vi "读取SuperDog数据.vi"(8 "length":u32=128, 9 "offset":u32, 10 "fileid":u32=65524, 11 "feature_id":u32=1) -> (1 "buffer out(Hex)":string, 2 "license handle":u32)   [LabVIEW 2009]
uses:
  dog_windows_UCPBI.dll
panel:
  out "function return 2":i32
  out "out handle":u32
  in  "vendor_code":string="Ur6fPGYDEBkws3SZISCrIAjySjKgu+8CGpfZwvGywxzzFI7qfH5o4nn4T/VCSRk/BzHd89oLkO1FSQ6hEVYUq6gMbLM2C/cFM+If39OR5tb8bGFz9qR0CZDkjzzjmu7KkZUG/Iybd++jcPT1fCPTGl6yJQ63DfZrtajYZMbIcHXXH5GeLmq0E8DxHQfjk36CNBnpZp3ut4e1U62BwqZI8PukpzjI2GcYs99UUUsufQbOliL2dlPu5jsionzy4pNB7CtL1sNOSyL4lXeGzFITSf8f2PBTMx9pRbZVpRKcaSkgwkYIgZXZK4Mh7WJhSM9dVyuowWAwHAuS1RiQbUqLqNZTlQihipkbiFrvlvM/xVR66Srt2LVSqv6RGu0aWaNM+SeJAKQlu1FskQm2TRpYQAGcH9IYTi3NGin13cji+Dth8rVwEY04N9GmpGLG1KBZxXFIIYBy0O8uMggrvjMlMgu9vg/saWFb+shkOQnET6WxlanEW2MfoWqVm2hwmy6exQBR69dptwkQ5qXprYd3dqA3rTyUqz4W29XJ+nztSzZRMl1Jt8sxCVvSX0Lg7SiRSoedaijV3a2EegSPrw4xW5o7O+yQItLwaVks4udB3kVz+wOrOTrxlWOz3u5MHdUzWFHlrTQRDlt9xBAqO+PT5M85/8ZLpyxHHIIpvOqXtCxgrtKMy1SD3O6zMZutZlcCE6Gj9CK6vz9O5JlMBBA5bEYYZSUUACDo9z6fP/F0VUeEMhqr9wsmyQdBIlBGlYM0GsvXLcJNL74RPewQkgLEhWc4txMcn6l0ey6Ic+qXpypp1e5qgjwyVACyJgZphW3HVcmpmld71etpUP0WgIY7Uuso2ZTDXKwBoh4l7Q5ZiKurwwQ5USgmL+vGx1H60ANV7LAoiEM2/cAiuUL+fKvyTMrWDED5hSzclM+TYLwc2vTgNmcQwlUcbjKlJIQTYSpPLpAa7xsThJ34yY5WOoiQLQ=="
  out "function return":i32
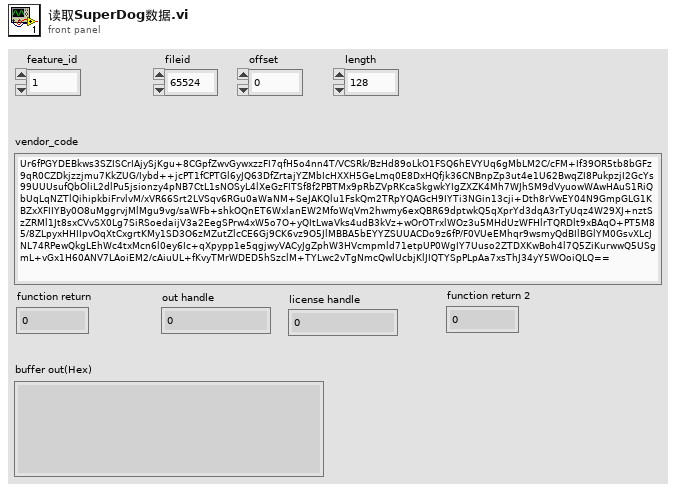
[diagram p1: front panel]
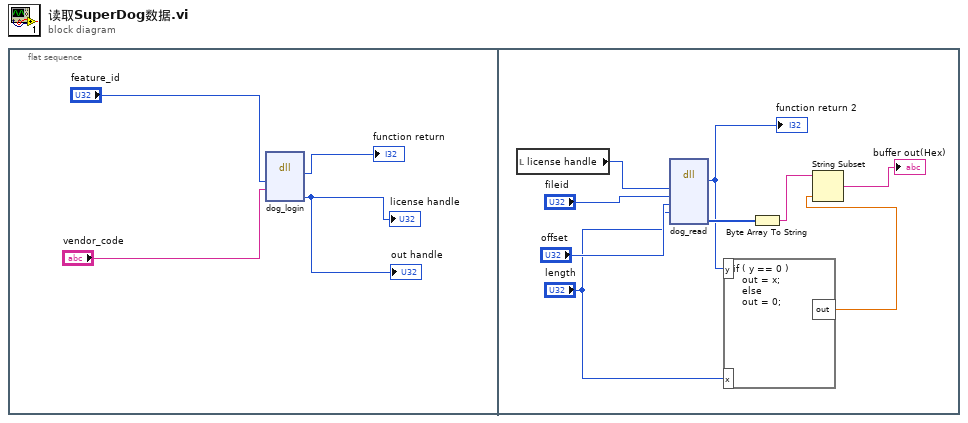
[diagram p0: block diagram]
diagram:
  n1 = flat-sequence {
    frame #0 {
      n2 = dll-call lib="E:/SubVI/SuperDog/dog_windows_UCPBI.dll" fn="dog_login"("feature_id"="feature_id", "vendor_code"="vendor_code") -> ("返回类型"=→"function return":u32, "out handle"=→"out handle" →"license handle":u32)  [unwired: 6 in, 2 out]
    }
    frame #1 {
      n3 = local read "license handle"() -> (w6:u32)
      n4 = dll-call lib="E:/SubVI/SuperDog/dog_windows_UCPBI.dll" fn="dog_read"("handle"=w6, "fileid"="fileid", "offset"="offset", "length"="length") -> ("返回类型"=w8:u32, "buffer"=w10:u8[])  [unwired: 8 in, 2 out]
      "function return 2" <- w8
      n5 = formula code="if ( y == 0 )\n   out = x;\n   else\n   out = 0;"("x"="length", "y"=w8) -> ("out"=w11:dbl)
      n6 = Byte Array To String(unsigned byte array=w10) -> (string=w9:string)
      n7 = String Subset(string=w9, length (rest)=w11) -> (substring=→"buffer out(Hex)":string)  [unwired: 1 in]
    }
  }
